vi "Read Data from Caller.vi"(7 "lv_icon.vi":refnum<vi>, 8 "error in (no error)":errorcluster, 10 "Default body text":T1 {"Body Text Spec"."Alignment" items=["left", "center", "right"]}, 11 "Init? (F)":bool) -> (0 "error out":errorcluster, 1 "Library Icon":picture, 2 "Icon Editor Invoker Type":T5, 3 "data":T4={"Text Visible?"=FALSE, "Text Opacity"=0, "Templ Visible?"=FALSE, "Templ Opacity"=0, "Relative Path from 1 to 2"=path "", "Image"=bytes[0], "All User Layers"=[], "Body Text"={"Line 1 text"="", "Line 2 text"="", "Line 3 text"="", "Line 4 text"="", "Line 1 color"=0, "Line 2 color"=0, "Line 3 color"=0, "Line 4 color"=0, "Body Text Spec"={"Font"="", "Alignment"=0, "Size"=3}, "Center text vertically"=FALSE, "Capitalize Text"=FALSE}} {"Body Text"."Body Text Spec"."Alignment" items=["left", "center", "right"]}, 4 "Valid?":bool, 5 "Valid Library icon?":bool)   [LabVIEW 2021]
uses:
  <resource>/plugins/IconEditor/Icon Editor Invoker Type.ctl
  <vilib>/LabVIEW Icon API/lv_icon/Controls/LabVIEW Icon Stored Information.ctl
  <vilib>/LabVIEW Icon API/lv_icon/Classes/Layer/Layer.lvclass
  <vilib>/LabVIEW Icon API/lv_icon/Controls/BodyText.ctl
  <vilib>/LabVIEW Icon API/lv_icon/Controls/Font.ctl
  <vilib>/LabVIEW Icon API/lv_icon/Controls/Alignment.ctl
  <vilib>/Utility/miscctls.llb/LVRectTypeDef.ctl
  <vilib>/LabVIEW Icon API/lv_icon/lv_icon.lvlib
panel:
  in  "String":string="Palette Icon"
  in  "Localized string":string="Icon Editor"
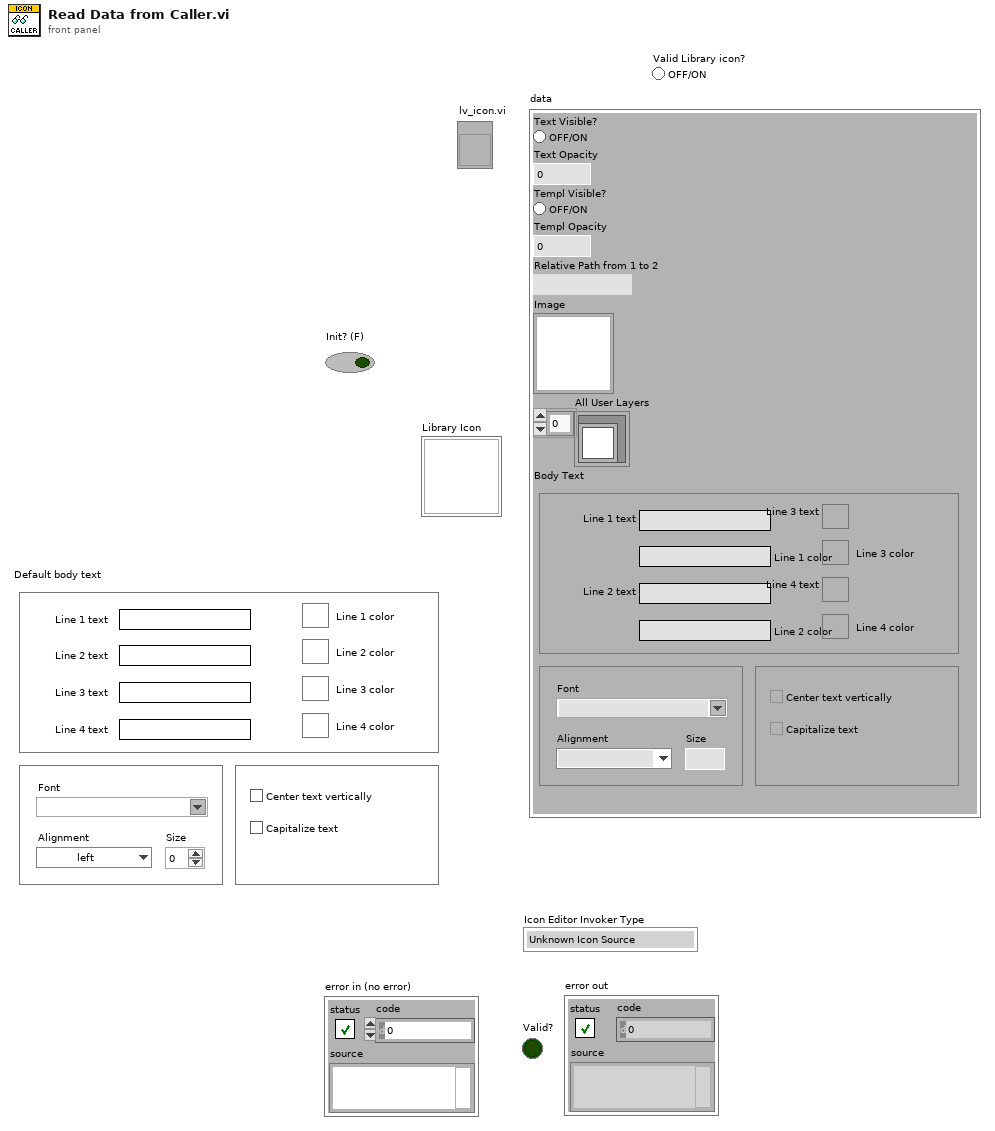
[diagram p1: front panel]
types:
  T1 = typedef "BodyText.ctl" = cluster{"Line 1 text":string, "Line 2 text":string, "Line 3 text":string, "Line 4 text":string, "Line 1 color":u32, "Line 2 color":u32, "Line 3 color":u32, "Line 4 color":u32, "Body Text Spec":cluster{"Font":T2, "Alignment":T3, "Size":u8}, "Center text vertically":bool, "Capitalize Text":bool}
  T2 = typedef "Font.ctl" = string
  T3 = typedef "Alignment.ctl" = u16
  T4 = typedef "LabVIEW Icon Stored Information.ctl" = cluster{"Text Visible?":bool, "Text Opacity":u8, "Templ Visible?":bool, "Templ Opacity":u8, "Relative Path from 1 to 2":path, "Image":picture, "All User Layers":refnum<class "Layer.lvclass">[], "Body Text":T1}
  T5 = typedef "Icon Editor Invoker Type.ctl" = enum32{"Unknown Icon Source", "VI Icon", "Library Icon (any library type)", "Palette icon", "Icon from App Method"}
  T6 = typedef "LVRectTypeDef.ctl" = cluster{"Left":i16, "Top":i16, "Right":i16, "Bottom":i16}
  T7 = typedef "Who Invoked Icon Editor.ctl" = cluster{"Icon Editor Invoker Type":T5, "App Refnum of Invoker":refnum<vi>, "Qualified Name of Invoker":string, "Path to Invoker":path}
  T8 = typedef "imagedata.ctl" = cluster{"image type":i32, "image depth":i32, "image":u8[], "mask":u8[], "colors":u32[], "Rectangle":cluster{"left":i16, "top":i16, "right":i16, "bottom":i16}}
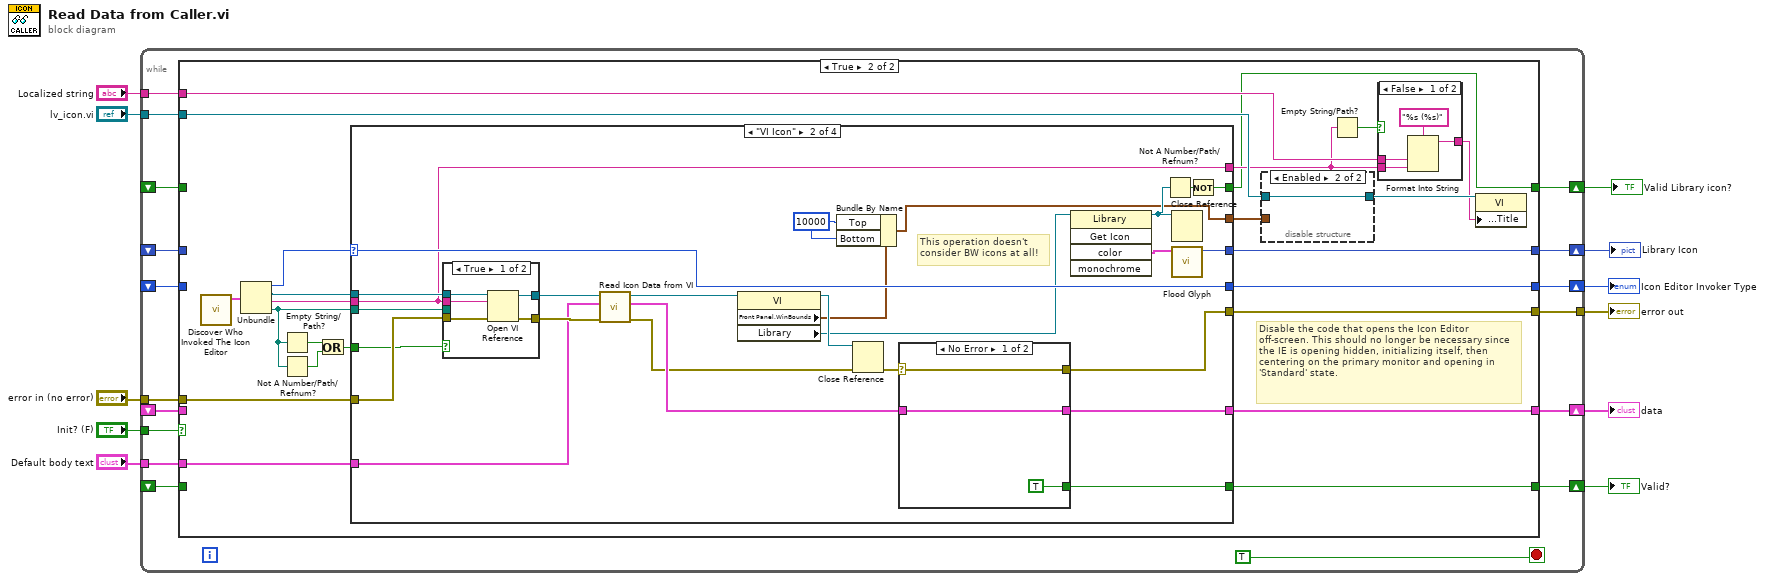
[diagram p0: block diagram]
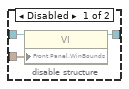
[diagram p3: hidden frame]
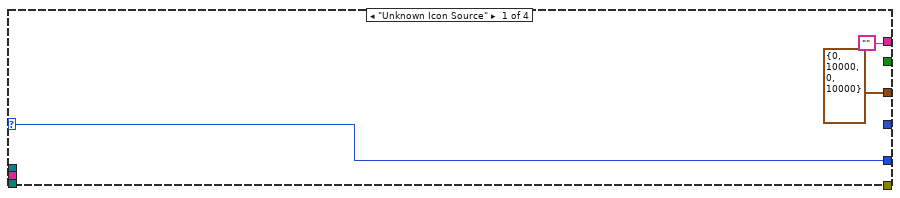
[diagram p5: hidden frame]
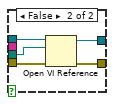
[diagram p6: hidden frame]
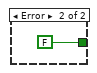
[diagram p7: hidden frame]
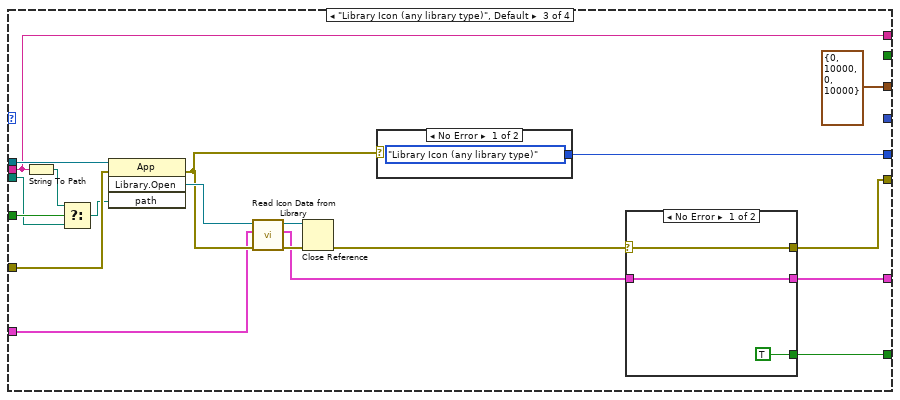
[diagram p8: hidden frame]
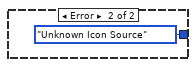
[diagram p9: hidden frame]
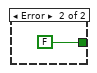
[diagram p10: hidden frame]
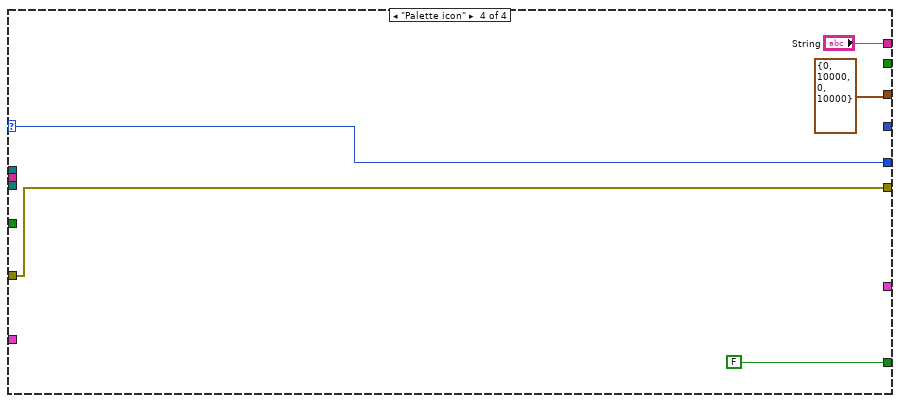
[diagram p11: hidden frame]
diagram:
  n1 = while {
    tunnel: [w28] -> w11
    tunnel: "error in (no error)" -> [w25]
    tunnel: "Init? (F)" -> [w24]
    tunnel: "lv_icon.vi" -> [w22]
    shift-right: [w23] -> w7
    shift-left: _ -> [w19]
    shift-right: [w26] -> w5
    shift-left: _ -> [w20]
    shift-right: [w27] -> w6
    shift-left: _ -> [w18]
    shift-right: [w17] -> w4
    shift-left: _ -> [w16]
    shift-right: [w15] -> w3
    shift-left: _ -> [w14]
    tunnel: "Default body text" -> [w13]
    tunnel: "Localized string" -> [w12]
    stop <- TRUE stop-if-true
    n2 = case shown="True" w24 {
      tunnel: [w31 w57] -> w28
      tunnel: [w34 w56] -> w26
      tunnel: [w32 w55] -> w27
      tunnel: w25 -> [w31 w54]
      tunnel: [w33 w50] -> w23
      tunnel: w22 -> [_ w41]
      tunnel: w20 -> [w34 _]
      tunnel: w19 -> [w33 _]
      tunnel: w18 -> [w32 _]
      tunnel: [w30 w44] -> w17
      tunnel: w16 -> [w30 _]
      tunnel: [w29 w35] -> w15
      tunnel: w14 -> [w29 _]
      tunnel: w13 -> [_ w43]
      tunnel: w12 -> [_ w42]
      frame False {
      }
      frame True {
        # "Disable the code that opens the Icon Editor off-screen. This should no longer be necessary since the IE is opening hidden, initializing itself, then centering on the primary monitor and opening in 'Standard' state."
        n3 = call <resource>:"Discover Who Invoked The Icon Editor.vi"() -> ("Who Invoked The Icon Editor?"=w53:T7)  [unwired: 11 out]
        n4 = Unbundle(w53) -> ("Icon Editor Invoker Type"=w51:T5, "App Refnum of Invoker"=w52:refnum<vi>, "Qualified Name of Invoker"=w46:string, "Path to Invoker"=w45:path)
        n5 = Empty String/Path?(string/path=w45) -> (empty?=w49:bool)
        n6 = Not A Number/Path/Refnum?(number/path/refnum=w45) -> (NaN/Path/Refnum?=w48:bool)
        n7 = Or(x=w49, y=w48) -> (x .or. y?=w47:bool)
        n8 = case shown="\"VI Icon\"" w51 {
          selector: w51 -> [w69 w86 _ w137]
          tunnel: [_ w92 w128 w138] -> w57
          tunnel: [_ w91 w127 _] -> w56
          tunnel: [_ w90 w126 FALSE] -> w55
          tunnel: w54 -> [_ w89 w125 w138]
          tunnel: w52 -> [_ w88 w119 _]
          tunnel: [w69 w86 w117 w137] -> w50
          tunnel: w46 -> [_ w70 w110 _]
          tunnel: w45 -> [_ w84 w115 _]
          tunnel: w47 -> [_ w85 w116 _]
          tunnel: [_ w76 _ _] -> w44
          tunnel: [_ w73 _ _] -> w35
          tunnel: w43 -> [_ w72 w112 _]
          tunnel: [T6 {"Left"=0, "Top"=10000, "Right"=0, "Bottom"=10000} ("Front Panel Window:Window Bounds") w71 T6 {"Left"=0, "Top"=10000, "Right"=0, "Bottom"=10000} ("Front Panel Window:Window Bounds") T6 {"Left"=0, "Top"=10000, "Right"=0, "Bottom"=10000} ("Front Panel Window:Window Bounds")] -> w40
          tunnel: ["" w70 w110 "String"] -> w36
          frame "Unknown Icon Source" {
          }
          frame "VI Icon" {
            w81 = i16 10000 ("left")
            # "This operation doesn't\nconsider BW icons at all!"
            n9 = case shown="True" w85 {
              tunnel: [w100 w105] -> w95
              tunnel: [w99 w104] -> w94
              tunnel: w89 -> [w98 w103]
              tunnel: w88 -> [w97 w102]
              tunnel: w70 -> [w96 _]
              tunnel: w84 -> [_ w101]
              frame True {
                n10 = Open VI Reference(application reference (local)=w97, vi path=w96, error in (no error)=w98) -> (vi reference=w100:refnum<vi>, error out=w99:errorcluster)  [unwired: 3 out]
              }
              frame False {
                n11 = Open VI Reference(application reference (local)=w102, vi path=w101, error in (no error)=w103) -> (vi reference=w105:refnum<vi>, error out=w104:errorcluster)  [unwired: 3 out]
              }
            }
            n12 = call <vilib>:"Read Icon Data from VI.vi"("error in (no error)"=w94, "Default body text"=w72, "VI Ref in"=w95) -> ("error out"=w80:errorcluster, "Data"=w87:T4, "VI Ref out"=w79:refnum<vi>)  [unwired: 6 in]
            n13 = property class="VI"(reference=w79) -> (reference out=w83:refnum<vi>, "Front Panel.WinBounds"=w82:T6, "Library"=w78:refnum<vi>)  [unwired: 1 in, 1 out]
            n14 = Bundle By Name(cluster=w82, "Top"=w81, "Bottom"=w81) -> (w71:T6)
            n15 = Close Reference(reference=w83, error in (no error)=w80) -> (error out=w93:errorcluster)
            n16 = case shown="No Error" w93 {
              selector: w93 -> [w108 _]
              tunnel: [w108 _] -> w92
              tunnel: [w106 _] -> w91
              tunnel: [TRUE FALSE] -> w90
              tunnel: w87 -> [w106 _]
              frame No Error {
              }
              frame Error {
              }
            }
            n17 = invoke class="Library" method="Get Icon"(reference=w78) -> (reference out=w75:refnum<vi>, "color"=w77:T8)  [unwired: 4 in, 3 out]
            n18 = Not A Number/Path/Refnum?(number/path/refnum=w75) -> (NaN/Path/Refnum?=w74:bool)
            n19 = Close Reference(reference=w75) -> ()  [unwired: 1 in, 1 out]
            n20 = call <vilib>:"Flood Glyph.vi"("image data"=w77) -> ("Pic Out"=w76:picture)  [unwired: 1 in, 9 out]
            n21 = Not(x=w74) -> (.not. x?=w73:bool)
          }
          frame "Library Icon (any library type)", Default {
            n22 = String To Path(string=w110) -> (path=w114:path)
            n23 = Select(t=w114, s=w116, f=w115) -> (s? t:f=w113:path)
            n24 = invoke class="App" method="Library.Open"(reference=w119, error in=w125, "path"=w113) -> (error out=w118:errorcluster, "Open Library"=w121:refnum<vi>)  [unwired: 1 in, 2 out]
            n25 = call <vilib>:"Read Icon Data from Library.vi"("error in (no error)"=w118, "Default body text"=w112, "Library in"=w121) -> ("error out"=w123:errorcluster, "Data"=w122:T4, "Library out"=w120:refnum<vi>)  [unwired: 6 in]
            n26 = Close Reference(reference=w120, error in (no error)=w123) -> (error out=w124:errorcluster)
            n27 = case shown="No Error" w118 {
              tunnel: [Icon_Editor_Invoker_Type."Library Icon (any library type)" ("Icon Editor Invoker Type") Icon_Editor_Invoker_Type."Unknown Icon Source" ("Icon Editor Invoker Type")] -> w117
              frame No Error {
              }
              frame Error {
              }
            }
            n28 = case shown="No Error" w124 {
              selector: w124 -> [w133 _]
              tunnel: [w133 _] -> w128
              tunnel: [w131 _] -> w127
              tunnel: [TRUE FALSE] -> w126
              tunnel: w122 -> [w131 _]
              frame No Error {
              }
              frame Error {
              }
            }
          }
          frame "Palette icon" {
          }
        }
        n29 = disable-structure shown="Enabled" {
          disable-tunnel: w41 -> [w60 w61]
          disable-tunnel: w40 -> [w59 _]
          disable-tunnel: [w58 w61] -> w39
          frame Disabled {
            n30 = property class="VI"(reference=w60, "Front Panel.WinBounds"=w59) -> (reference out=w58:refnum<vi>)  [unwired: 1 in, 1 out]
          }
          frame Enabled {
          }
        }
        n31 = Empty String/Path?(string/path=w36) -> (empty?=w37:bool)
        n32 = case shown="False" w37 {
          tunnel: w42 -> [w65 w66]
          tunnel: w36 -> [w63 _]
          tunnel: [w62 w66] -> w38
          frame False {
            n33 = Format Into String(format string="%s (%s)", w65, w63) -> (resulting string=w62:string)  [unwired: 2 in, 1 out]
          }
          frame True {
          }
        }
        n34 = property class="VI"(reference=w39, "Front Panel.Title"=w38) -> ()  [unwired: 1 in, 2 out]
      }
    }
  }
  "error out" <- w11
  "Valid?" <- w6
  "Icon Editor Invoker Type" <- w7
  "data" <- w5
  "Library Icon" <- w4
  "Valid Library icon?" <- w3
